vi "AlliGator Get Phase Lifetime & Phasor Ratio at Pixel.vi"(8 "error in (no error)":errorcluster, 9 "Intensity (F)/Amplitude (T) weighted":bool, 10 "Phasor Frequency":dbl[unit], 11 "Phasor":csg) -> (0 "error out":errorcluster, 1 "Phasor/Amplitude Ratio":dbl, 2 "Phasor Ratio Plot Name Suffix":string, 3 "Phase Lifetime":dbl[unit])   [LabVIEW 2021, in "AlliGator Image Profile Window.lvlib"]
doc: "Computes Phase Lifetime and Phasor Ratio."
uses:
  AlliGator Image Profile Window.lvlib
  Phasor/Phasor.lvlib
  Phasor Ratio/AlliGator Phasor Ratio.lvlib
panel:
  # "see the AlliGator License on the block diagram (Ctrl+E or Window:Show Block Diagram)"
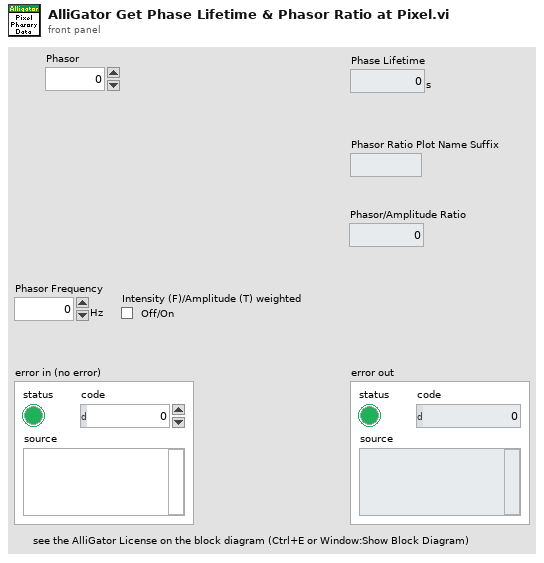
[diagram p1: front panel]
types:
  T1 = typedef "Phasor.lvlib/Phasor (g, s).ctl" = cluster{"g":dbl, "s":dbl}
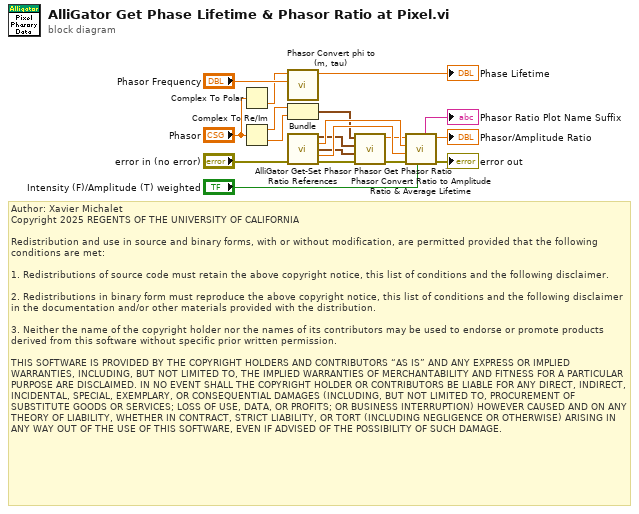
[diagram p0: block diagram]
diagram:
  # "Author: Xavier Michalet\nCopyright 2025 REGENTS OF THE UNIVERSITY OF CALIFORNIA\n\nRedistribution and use in source and binary forms, with or without modification, are permitted provided that the following conditions are met:\n\n1. Redistributions of source code must retain the above copyright notice, this list of conditions and the following disclaimer.\n\n2. Redistributions in binary form must reproduce the above copyright notice, this list of conditions and the following disclaimer in the documentation and/or other materials provided with the distribution.\n\n3. Neither the name of the copyright holder nor the names of its contributors may be used to endorse or promote products derived from this software without specific prior written permission.\n\nTHIS SOFTWARE IS PROVIDED BY THE COPYRIGHT HOLDERS AND CONTRIBUTORS “AS IS” AND ANY EXPRESS OR IMPLIED WARRANTIES, INCLUDING, BUT NOT LIMITED TO, THE IMPLIED WARRANTIES OF MERCHANTABILITY AND FITNESS FOR A PARTICULAR PURPOSE ARE DISCLAIMED. IN NO EVENT SHALL THE COPYRIGHT HOLDER OR CONTRIBUTORS BE LIABLE FOR ANY DIRECT, INDIRECT, INCIDENTAL, SPECIAL, EXEMPLARY, OR CONSEQUENTIAL DAMAGES (INCLUDING, BUT NOT LIMITED TO, PROCUREMENT OF SUBSTITUTE GOODS OR SERVICES; LOSS OF USE, DATA, OR PROFITS; OR BUSINESS INTERRUPTION) HOWEVER CAUSED AND ON ANY THEORY OF LIABILITY, WHETHER IN CONTRACT, STRICT LIABILITY, OR TORT (INCLUDING NEGLIGENCE OR OTHERWISE) ARISING IN ANY WAY OUT OF THE USE OF THIS SOFTWARE, EVEN IF ADVISED OF THE POSSIBILITY OF SUCH DAMAGE."
  n1 = Complex To Polar(r * e^(i*theta)="Phasor") -> (theta=w2:sgl)  [unwired: 1 out]
  n2 = Complex To Re/Im(x + iy="Phasor") -> (x=w9:sgl, y=w10:sgl)
  n3 = call "Phasor Convert phi to (m, tau).vi"("Phasor Frequency"="Phasor Frequency", "Phase"=w2) -> ("Phase Lifetime"=→"Phase Lifetime":dbl[unit])  [unwired: 8 in, 1 out]
  n4 = Bundle(w9, w10) -> (w11:cluster{sgl, sgl})  [unwired: 1 in]
  n5 = call "AlliGator Get-Set Phasor Ratio References.vi"("error in (no error)"="error in (no error)") -> ("Reference Phasor 1"=w6:T1, "Reference Lifetime 1"=w16:dbl[unit], "Reference Phasor 2"=w5:T1, "Reference Lifetime 2"=w17:dbl[unit], "error out"=w15:errorcluster)  [unwired: 7 in, 3 out]
  n6 = call "Phasor Get Phasor Ratio.vi"("Error In"=w15, "Reference Phasor 2"=w5, "Reference Phasor 1"=w6, "Phasor"=w11) -> ("Error Out"=w8:errorcluster, "Phasor Ratio (f1)"=w7:dbl)  [unwired: 5 in, 1 out]
  n7 = call "Phasor Convert Ratio to Amplitude Ratio & Average Lifetime.vi"("Compute Amplitude Ratio"="Intensity (F)/Amplitude (T) weighted", "error in (no error)"=w8, "Reference Lifetime 2"=w17, "Reference Lifetime 1"=w16, "Phasor Ratio (f1)"=w7) -> ("error out"=→"error out":errorcluster, "Phasor/Amplitude Ratio"=→"Phasor/Amplitude Ratio":dbl, "Phasor Ratio Plot Name Suffix"=→"Phasor Ratio Plot Name Suffix":string)  [unwired: 2 in, 2 out]
